vi "SettingsDatabase--Old Interface Glue.vi"(11 "Response":T5) -> (1 "Funnel Properties":T6[](array[typedef]) {"Direction" items=["Forward", "Backward"]}, 2 "Rectangle Properties":T10[](array[typedef]) {"Fill Orientation" items=["Horizontal", "Vertical", ""]; "Direction" items=["Forward", "Backward"]}, 3 "Path Properties":T11[](array[typedef]) {"Fill Orientation" items=["Horizontal", "Vertical", ""]; "Direction" items=["Forward", "Backward"]})   [LabVIEW 2019]
uses:
  subVIs/typedefs/Path Properties - cluster.ctl
  subVIs/typedefs/Voltage - cluster.ctl
  subVIs/typedefs/Schedule - enum.ctl
  <userlib>/LevyLab/Relay Box/Typedefs/Resistor--enum.ctl
  subVIs/typedefs/Rectangle Properties - cluster.ctl
  subVIs/typedefs/Funnel Properties - cluster.ctl
  Typedefs/PublicEvents--Setting Database.PathsUpdated.ctl
  Path Settings/Path Settings.lvclass
  C:/Users/Albro/Documents/GitHub/AFM-Lithography/lvsrc/Classes/Settings/ObjectSettings/ObjectSettings.lvclass
  Typedefs/PublicEvents--Setting Database.RectanglesUpdated.ctl
  Rectangle Settings/Rectangle Settings.lvclass
  Typedefs/PublicEvents--Setting Database.FunnelsUpdated.ctl
  Funnel Settings/Funnel Settings.lvclass
  Typedefs/PublicEvents--Setting Database.DotsUpdated.ctl
  Dot Settings/Dot Settings.lvclass
  ObjectSettings/ObjectSettings.lvclass/ObjectSettings.ctl
  Funnel Settings/Funnel Settings.lvclass/Funnel Settings.ctl
  Rectangle Settings/Rectangle Settings.lvclass/Rectangle Settings.ctl
  Path Settings/Path Settings.lvclass/Path Settings.ctl
  ObjectSettings/Accessors/Read Direction.vi
  ObjectSettings/Accessors/Read Enabled.vi
  ObjectSettings/Accessors/Read Speed.vi
  ObjectSettings/Accessors/Read Voltage.vi
  Funnel Settings/Accessors/Read Bottom Segments.vi
  Funnel Settings/Accessors/Read Smooth Segments.vi
  ObjectSettings/Accessors/Read Resistance.vi
  Rectangle Settings/Accessors/Read Fill Orientation.vi
  Rectangle Settings/Accessors/Read Fill Spacing.vi
  Path Settings/Accessors/Read Fill Orientation.vi
  Path Settings/Accessors/Read Fill Spacing.vi
  Path Settings/Accessors/Read Interpolation.vi
  Path Settings/Accessors/Read Smooth Segments.vi
  <userlib>/LevyLab/Relay Box/Relay-Box.lvclass
  Setting Database.lvclass
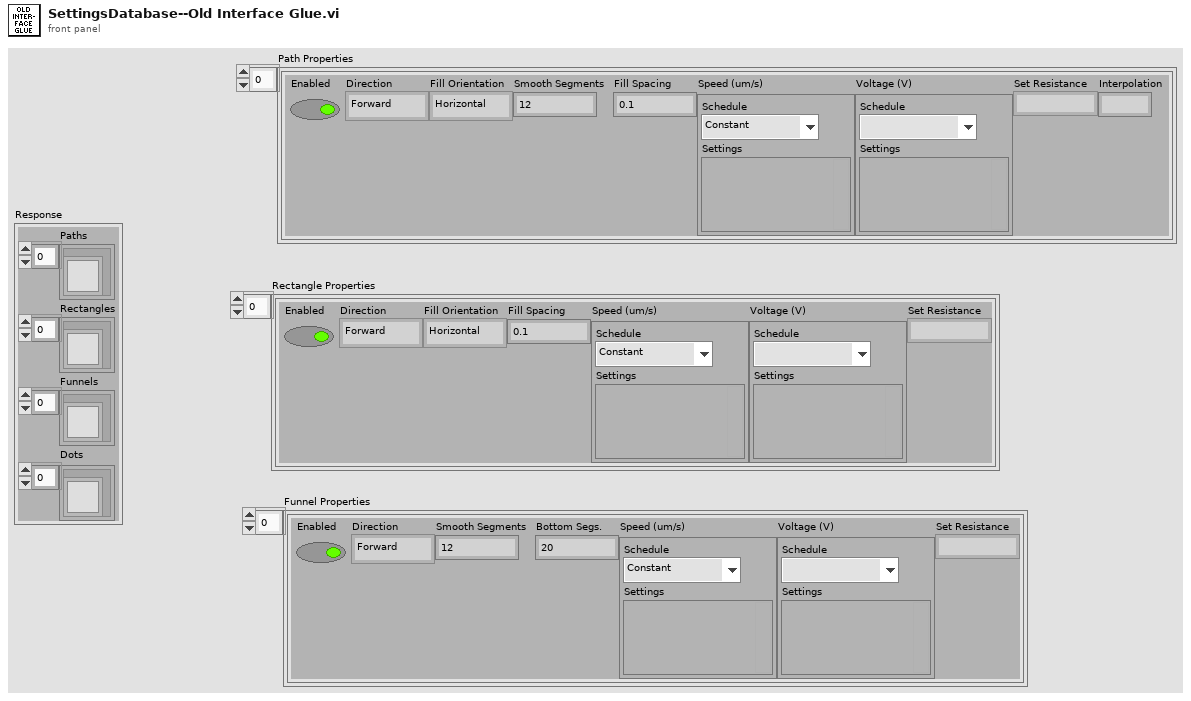
[diagram p1: front panel]
types:
  T1 = typedef "Setting Database.lvclass/PublicEvents--Setting Database.PathsUpdated.ctl" = refnum<class "Path Settings.lvclass">[]
  T2 = typedef "Setting Database.lvclass/PublicEvents--Setting Database.RectanglesUpdated.ctl" = refnum<class "Rectangle Settings.lvclass">[]
  T3 = typedef "Setting Database.lvclass/PublicEvents--Setting Database.FunnelsUpdated.ctl" = refnum<class "Funnel Settings.lvclass">[]
  T4 = typedef "Setting Database.lvclass/PublicEvents--Setting Database.DotsUpdated.ctl" = refnum<class "Dot Settings.lvclass">[]
  T5 = cluster{"Paths":T1, "Rectangles":T2, "Funnels":T3, "Dots":T4}
  T6 = typedef "Funnel Properties - cluster.ctl" = cluster{"Enabled":bool, "Direction":u16, "Smooth Segments":dbl, "Bottom Segs.":dbl, "Speed (um/s)":T7, "Voltage (V)":T7, "Set Resistance":T9}
  T7 = typedef "Voltage - cluster.ctl" = cluster{"Schedule":T8, "Settings":variant}
  T8 = typedef "Schedule - enum.ctl" = enum16{"Constant", "Ramp", "Fn. Generator", "Formula"}
  T9 = typedef "Relay-Box.lvclass/Resistor--enum.ctl" = enum16{"open", "discharge tip", "0 ohms", "100k ohm", "10M ohm", "1G ohm"}
  T10 = typedef "Rectangle Properties - cluster.ctl" = cluster{"Enabled":bool, "Direction":u16, "Fill Orientation":u16, "Fill Spacing":dbl, "Speed (um/s)":T7, "Voltage (V)":T7, "Set Resistance":T9}
  T11 = typedef "Path Properties - cluster.ctl" = cluster{"Enabled":bool, "Direction":u16, "Fill Orientation":u16, "Smooth Segments":dbl, "Fill Spacing":dbl, "Speed (um/s)":T7, "Voltage (V)":T7, "Set Resistance":T9, "Interpolation":dbl}
  T12 = enum16{"Open", "Discharge Tip", "0 ohm", "100 kohm", "10 Mohm", "1 Gohm"}
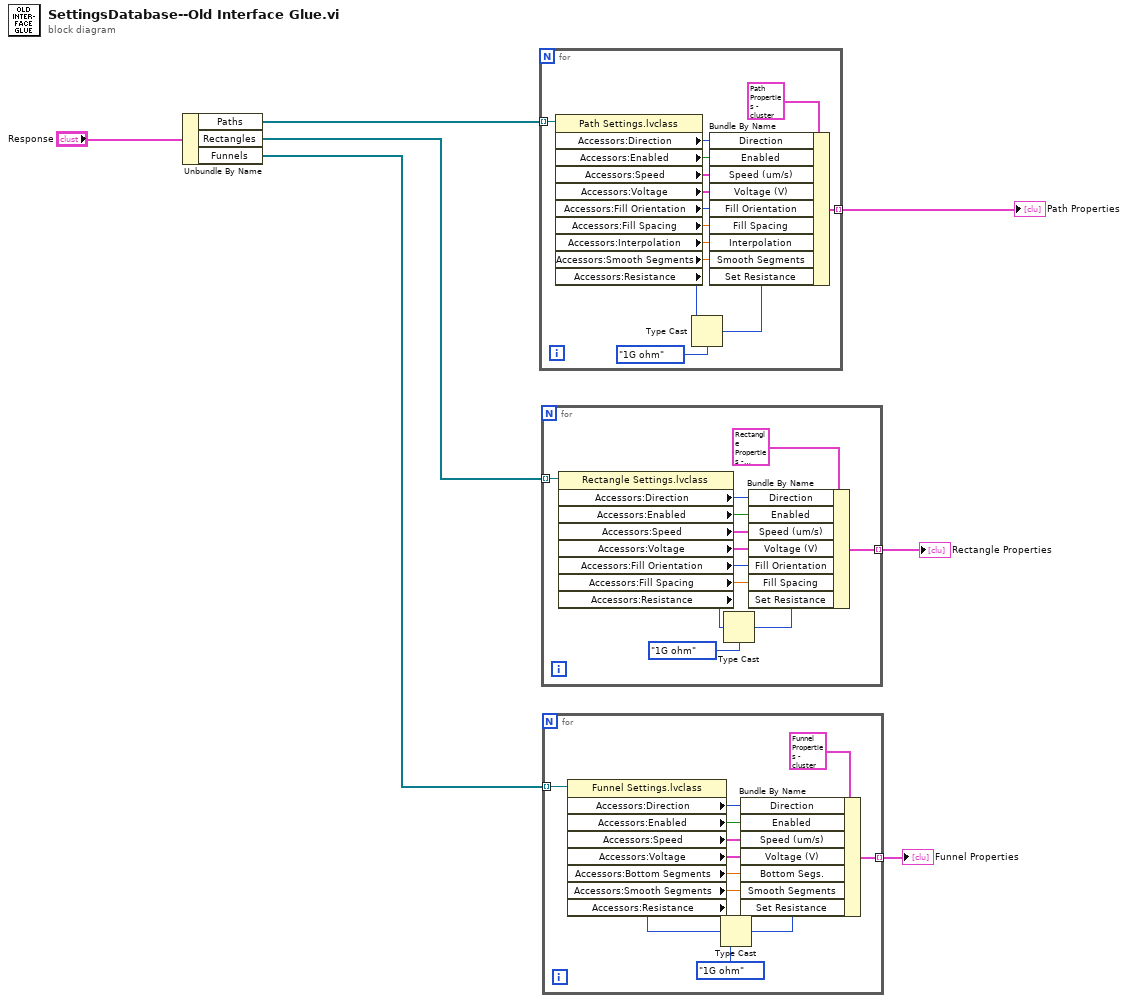
[diagram p0: block diagram]
diagram:
  n1 = Unbundle By Name("Response") -> ("Paths"=w7:T1, "Rectangles"=w5:T2, "Funnels"=w3:T3)
  n2 = for {
    tunnel: w7 -> [w20] mode=indexing
    tunnel: [w11] -> w6 mode=indexing
    n3 = property class="Path Settings.lvclass"(reference=w20) -> ("Accessors:Direction"=w19:u16, "Accessors:Enabled"=w18:bool, "Accessors:Speed"=w17:cluster{"Schedule":u16, "Settings":variant}, "Accessors:Voltage"=w16:cluster{"Schedule":u16, "Settings":variant}, "Accessors:Fill Orientation"=w15:u16, "Accessors:Fill Spacing"=w14:dbl, "Accessors:Interpolation"=w13:dbl, "Accessors:Smooth Segments"=w12:dbl, "Accessors:Resistance"=w9:T12)  [unwired: 1 in, 2 out]
    n4 = Type Cast(type=Resistor--enum."1G ohm" ("Set Resistance"), x=w9) -> (*(type *) &x=w8:T9)
    n5 = Bundle By Name(cluster=T11 {"Enabled"=TRUE, "Direction"=0, "Fill Orientation"=0, "Smooth Segments"=12.0, "Fill Spacing"=0.1, "Speed (um/s)"={"Schedule"=enum."Constant", "Settings"=variant(dbl 10.0)}, "Voltage (V)"={"Schedule"=enum."Constant", "Settings"=variant(dbl 10.0)}, "Set Resistance"=enum."1G ohm", "Interpolation"=0.1} ("Path Property"), "Direction"=w19, "Enabled"=w18, "Speed (um/s)"=w17, "Voltage (V)"=w16, "Fill Orientation"=w15, "Fill Spacing"=w14, "Interpolation"=w13, "Smooth Segments"=w12, "Set Resistance"=w8) -> (w11:T11)
  }
  "Path Properties" <- w6
  n6 = for {
    tunnel: w5 -> [w33] mode=indexing
    tunnel: [w26] -> w4 mode=indexing
    n7 = property class="Rectangle Settings.lvclass"(reference=w33) -> ("Accessors:Direction"=w32:u16, "Accessors:Enabled"=w31:bool, "Accessors:Speed"=w30:cluster{"Schedule":u16, "Settings":variant}, "Accessors:Voltage"=w29:cluster{"Schedule":u16, "Settings":variant}, "Accessors:Fill Orientation"=w28:u16, "Accessors:Fill Spacing"=w27:dbl, "Accessors:Resistance"=w23:T12)  [unwired: 1 in, 2 out]
    n8 = Type Cast(type=Resistor--enum."1G ohm" ("Set Resistance"), x=w23) -> (*(type *) &x=w22:T9)
    n9 = Bundle By Name(cluster=T10 {"Enabled"=FALSE, "Direction"=0, "Fill Orientation"=0, "Fill Spacing"=0.0, "Speed (um/s)"={"Schedule"=enum."Constant", "Settings"=variant}, "Voltage (V)"={"Schedule"=enum."Constant", "Settings"=variant}, "Set Resistance"=enum."open"} ("Rectangle Property"), "Direction"=w32, "Enabled"=w31, "Speed (um/s)"=w30, "Voltage (V)"=w29, "Fill Orientation"=w28, "Fill Spacing"=w27, "Set Resistance"=w22) -> (w26:T10)
  }
  "Rectangle Properties" <- w4
  n10 = for {
    tunnel: w3 -> [w45] mode=indexing
    tunnel: [w38] -> w2 mode=indexing
    n11 = property class="Funnel Settings.lvclass"(reference=w45) -> ("Accessors:Direction"=w44:u16, "Accessors:Enabled"=w43:bool, "Accessors:Speed"=w42:cluster{"Schedule":u16, "Settings":variant}, "Accessors:Voltage"=w41:cluster{"Schedule":u16, "Settings":variant}, "Accessors:Bottom Segments"=w40:dbl, "Accessors:Smooth Segments"=w39:dbl, "Accessors:Resistance"=w35:T12)  [unwired: 1 in, 2 out]
    n12 = Type Cast(type=Resistor--enum."1G ohm" ("Set Resistance"), x=w35) -> (*(type *) &x=w34:T9)
    n13 = Bundle By Name(cluster=T6 {"Enabled"=FALSE, "Direction"=0, "Smooth Segments"=0.0, "Bottom Segs."=0.0, "Speed (um/s)"={"Schedule"=enum."Constant", "Settings"=variant}, "Voltage (V)"={"Schedule"=enum."Constant", "Settings"=variant}, "Set Resistance"=enum."open"} ("Funnel Property"), "Direction"=w44, "Enabled"=w43, "Speed (um/s)"=w42, "Voltage (V)"=w41, "Bottom Segs."=w40, "Smooth Segments"=w39, "Set Resistance"=w34) -> (w38:T6)
  }
  "Funnel Properties" <- w2
